vi "setExposure.vi"(11 "Exposure Time (s)":sgl=0.01 step=0.001 format="%.4f") -> ()   [LabVIEW 2016]
uses:
  variables/imageSettings.vi
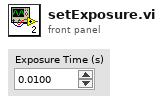
[diagram p1: front panel]
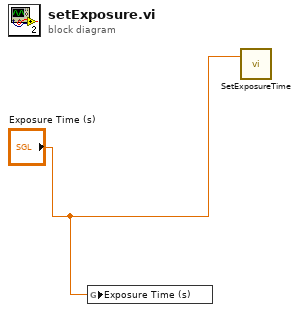
[diagram p0: block diagram]
diagram:
  n1 = global write "imageSettings.vi" "Exposure Time (s)"("Exposure Time (s)") -> ()
  n2 = call <userlib>:"SetExposureTime.vi"("time"="Exposure Time (s)") -> ()  [unwired: 1 in, 2 out]
